vi "Initialize Stored Session.vi"(8 "error in (no error)":errorcluster, 11 "Client ID":string) -> (0 "error out":errorcluster)   [LabVIEW 2013, in "MQTT Server.lvlib" / "StoredSessions.lvclass"]
uses:
  StoredSessions.lvclass
  Session State -- cluster.ctl
  <vilib>/LabVIEW Open Source Project/MQTT Control Packets/Control Packets/SUBSCRIBE/Topic Subscription -- cluster.ctl
  <vilib>/LabVIEW Open Source Project/MQTT Control Packets/Control Packets/ControlPacket/QualityOfService -- enum.ctl
  <vilib>/LabVIEW Open Source Project/MQTT Control Packets/Control Packets/ControlPacket/ControlPacket.lvclass
  <vilib>/LabVIEW Open Source Project/MQTT Control Packets/Control Packets/SUBSCRIBE/SUBSCRIBE.lvclass
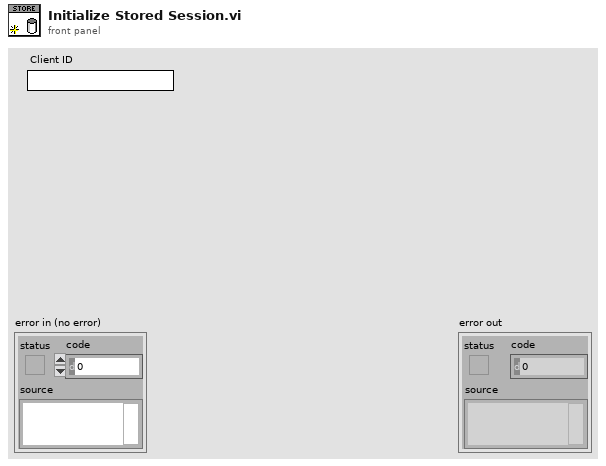
[diagram p1: front panel]
types:
  T1 = typedef "MQTT Server.lvlib/StoredSessions.lvclass/Session State -- cluster.ctl" = cluster{"Client ID":string, "Subscriptions":T2[], "PUBREC":u16[]}
  T2 = typedef "MQTT_Control_Packets.lvlib/SUBSCRIBE.lvclass/Topic Subscription -- cluster.ctl" = cluster{"Topic Filter":string, "QoS":T3}
  T3 = typedef "MQTT_Control_Packets.lvlib/ControlPacket.lvclass/QualityOfService -- enum.ctl" = enum16{"0 (At Most Once)", "1 (At Least Once)", "2 (Exactly Once)"}
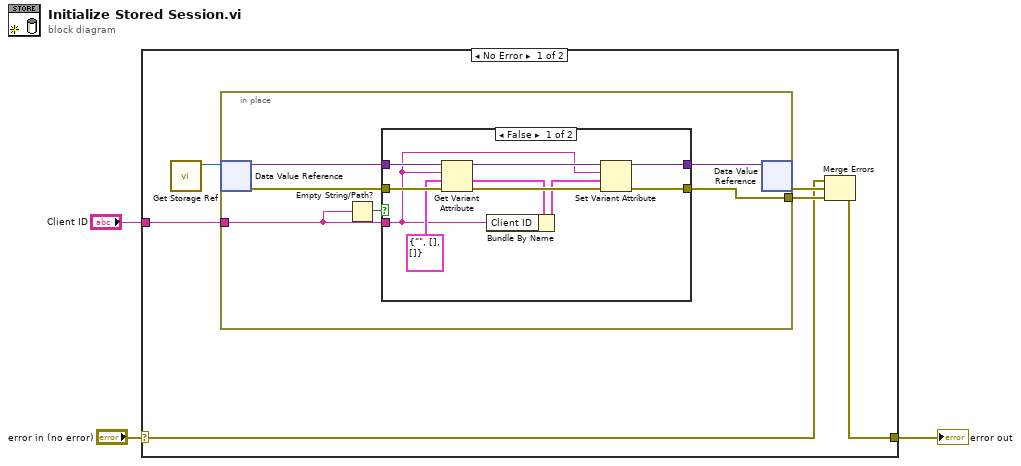
[diagram p0: block diagram]
diagram:
  n1 = case shown="No Error" "error in (no error)" {
    selector: "error in (no error)" -> [w6 w28]
    tunnel: [w5 w28] -> w2
    tunnel: "Client ID" -> [w4 _]
    frame No Error {
      n2 = call "Get Storage Ref.vi"() -> ("Storage"=w9:refnum<data-value>)  [unwired: 11 in]
      n3 = in-place {
        in-place-border: [w13] -> w8
        in-place-border: w4 -> [w10]
        n4 = in-place-dvr #1(w9) -> (w15:variant, w12:errorcluster)
        n5 = Empty String/Path?(string/path=w10) -> (empty?=w11:bool)
        n6 = case shown="False" w11 {
          tunnel: w15 -> [w25 w27]
          tunnel: [w22 w27] -> w14
          tunnel: [w19 w26] -> w13
          tunnel: w12 -> [w24 w26]
          tunnel: w10 -> [w16 _]
          frame False {
            n7 = Get Variant Attribute(Variant=w25, name=w16, default value (empty Variant)=T1 {"Client ID"="", "Subscriptions"=[], "PUBREC"=[]} ("Stored Session"), error in=w24) -> (duplicate Variant=w23:variant, value=w18:T1, error out=w20:errorcluster)  [unwired: 1 out]
            n8 = Bundle By Name(cluster=w18, "Client ID"=w16) -> (w17:T1)
            n9 = Set Variant Attribute(Variant=w23, name=w16, value=w17, error in=w20) -> (Variant out=w22:variant, error out=w19:errorcluster)  [unwired: 1 out]
          }
          frame True {
          }
        }
        n10 = in-place-dvr #1(w14) -> (w7:errorcluster)  [unwired: 1 out]
      }
      n11 = Merge Errors(w6, w7, w8) -> (w5:errorcluster)
    }
    frame Error {
    }
  }
  "error out" <- w2
